vi "NameAllGraph.vi"(9 "channelNames 2":refnum<vi>[](array[refnum]), 10 "showAll array":refnum<vi>[](array[refnum]), 11 "WaveformGraph in":refnum<vi>) -> ()   [LabVIEW 2013]
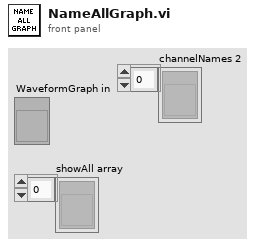
[diagram p1: front panel]
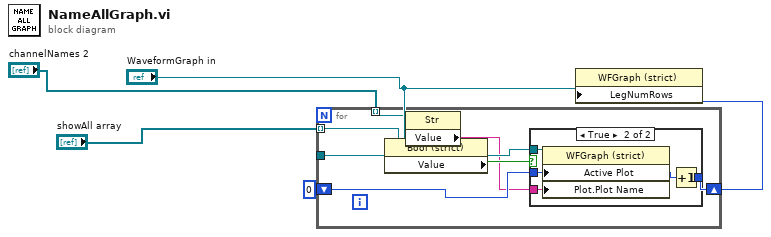
[diagram p0: block diagram]
diagram:
  n1 = for {
    tunnel: "WaveformGraph in" -> [w12]
    tunnel: "showAll array" -> [w11] mode=indexing
    shift-right: [w9] -> w4
    shift-left: i8 0 -> [w8]
    tunnel: "channelNames 2" -> [w7] mode=indexing
    n2 = property class="Bool (strict)"(reference=w11) -> ("Value"=w10:bool)  [unwired: 1 in, 2 out]
    n3 = property class="Str"(reference=w7) -> ("Value"=w6:string)  [unwired: 1 in, 2 out]
    n4 = case shown="True" w10 {
      tunnel: w12 -> [_ w17]
      tunnel: w8 -> [w13 w14]
      tunnel: w6 -> [_ w16]
      tunnel: [w13 w15] -> w9
      frame False {
      }
      frame True {
        n5 = property class="WFGraph (strict)"(reference=w17, "Active Plot"=w14, "Plot.Plot Name"=w16) -> ()  [unwired: 1 in, 2 out]
        n6 = Increment(x=w14) -> (x+1=w15:i8)
      }
    }
  }
  n7 = property class="WFGraph (strict)"(reference="WaveformGraph in", "LegNumRows"=w4) -> ()  [unwired: 1 in, 2 out]
